vi "Integer CompareTo.vi"(10 "input 2":i32, 11 "input 1":i32) -> (3 "comparison":i32)   [LabVIEW 2015, in "Chassis TimeSync System Explorer.lvlib"]
uses:
  Chassis TimeSync System Explorer.lvlib
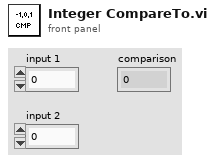
[diagram p1: front panel]
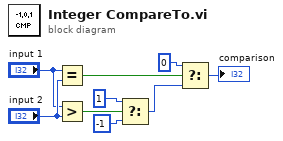
[diagram p0: block diagram]
diagram:
  n1 = Equal?(x="input 1", y="input 2") -> (x = y?=w2:bool)
  n2 = Greater?(x="input 1", y="input 2") -> (0:w4:bool)
  n3 = Select(t=1, s=w4, f=-1) -> (s? t:f=w3:i32)
  n4 = Select(t=0, s=w2, f=w3) -> (s? t:f=→"comparison":i32)
